vi "comport.vi"() -> ()   [LabVIEW 2022 SP3]
panel:
  in  "COM 6":string
  in  "Refresh Button":bool
  in  "COM 5":string
  in  "COM 4":string
  in  "COM 3":string
  in  "COM 2":string
  out "error out 8":errorcluster
  out "error out 7":errorcluster
  out "error out 6":errorcluster
  out "error out 5":errorcluster
  out "error out 4":errorcluster
  out "error out 3":errorcluster
  out "error out 2":errorcluster
  in  "OK Button":bool
  out "error out":errorcluster
  in  "3":string
  in  "2":string
  in  "1":string
  in  "COM":string
  # "REFERENCE CHECK"
  # "COM A"
  # "COM B"
  # "COM C"
  # "COM D"
  # "Refresh"
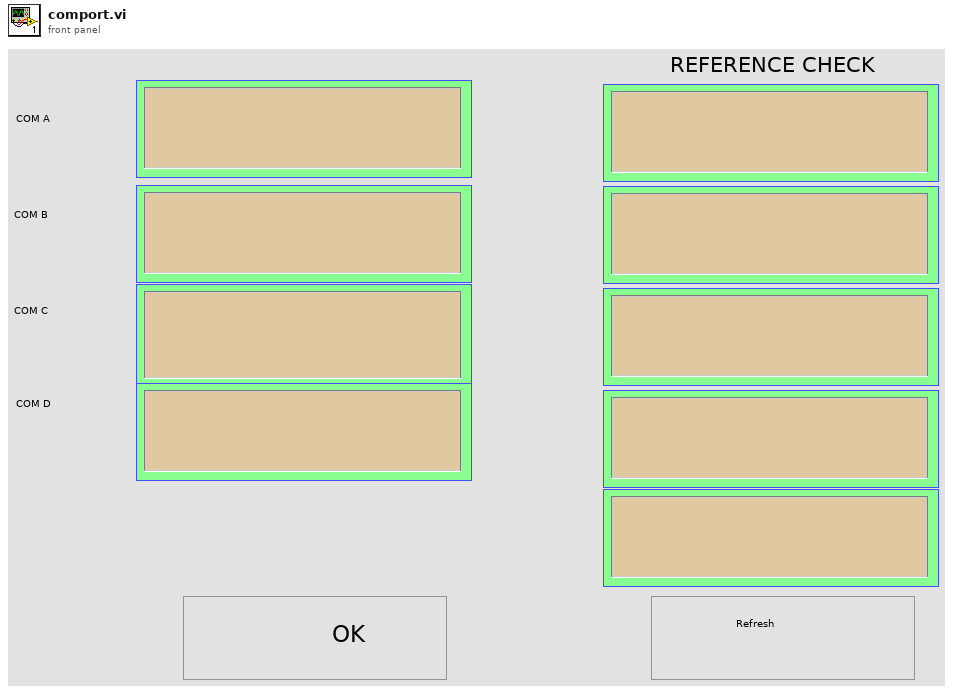
[diagram p1: front panel]
types:
  T1 = enum16{"open", "replace", "create", "open or create", "replace or create", "replace or create with confirmation"}
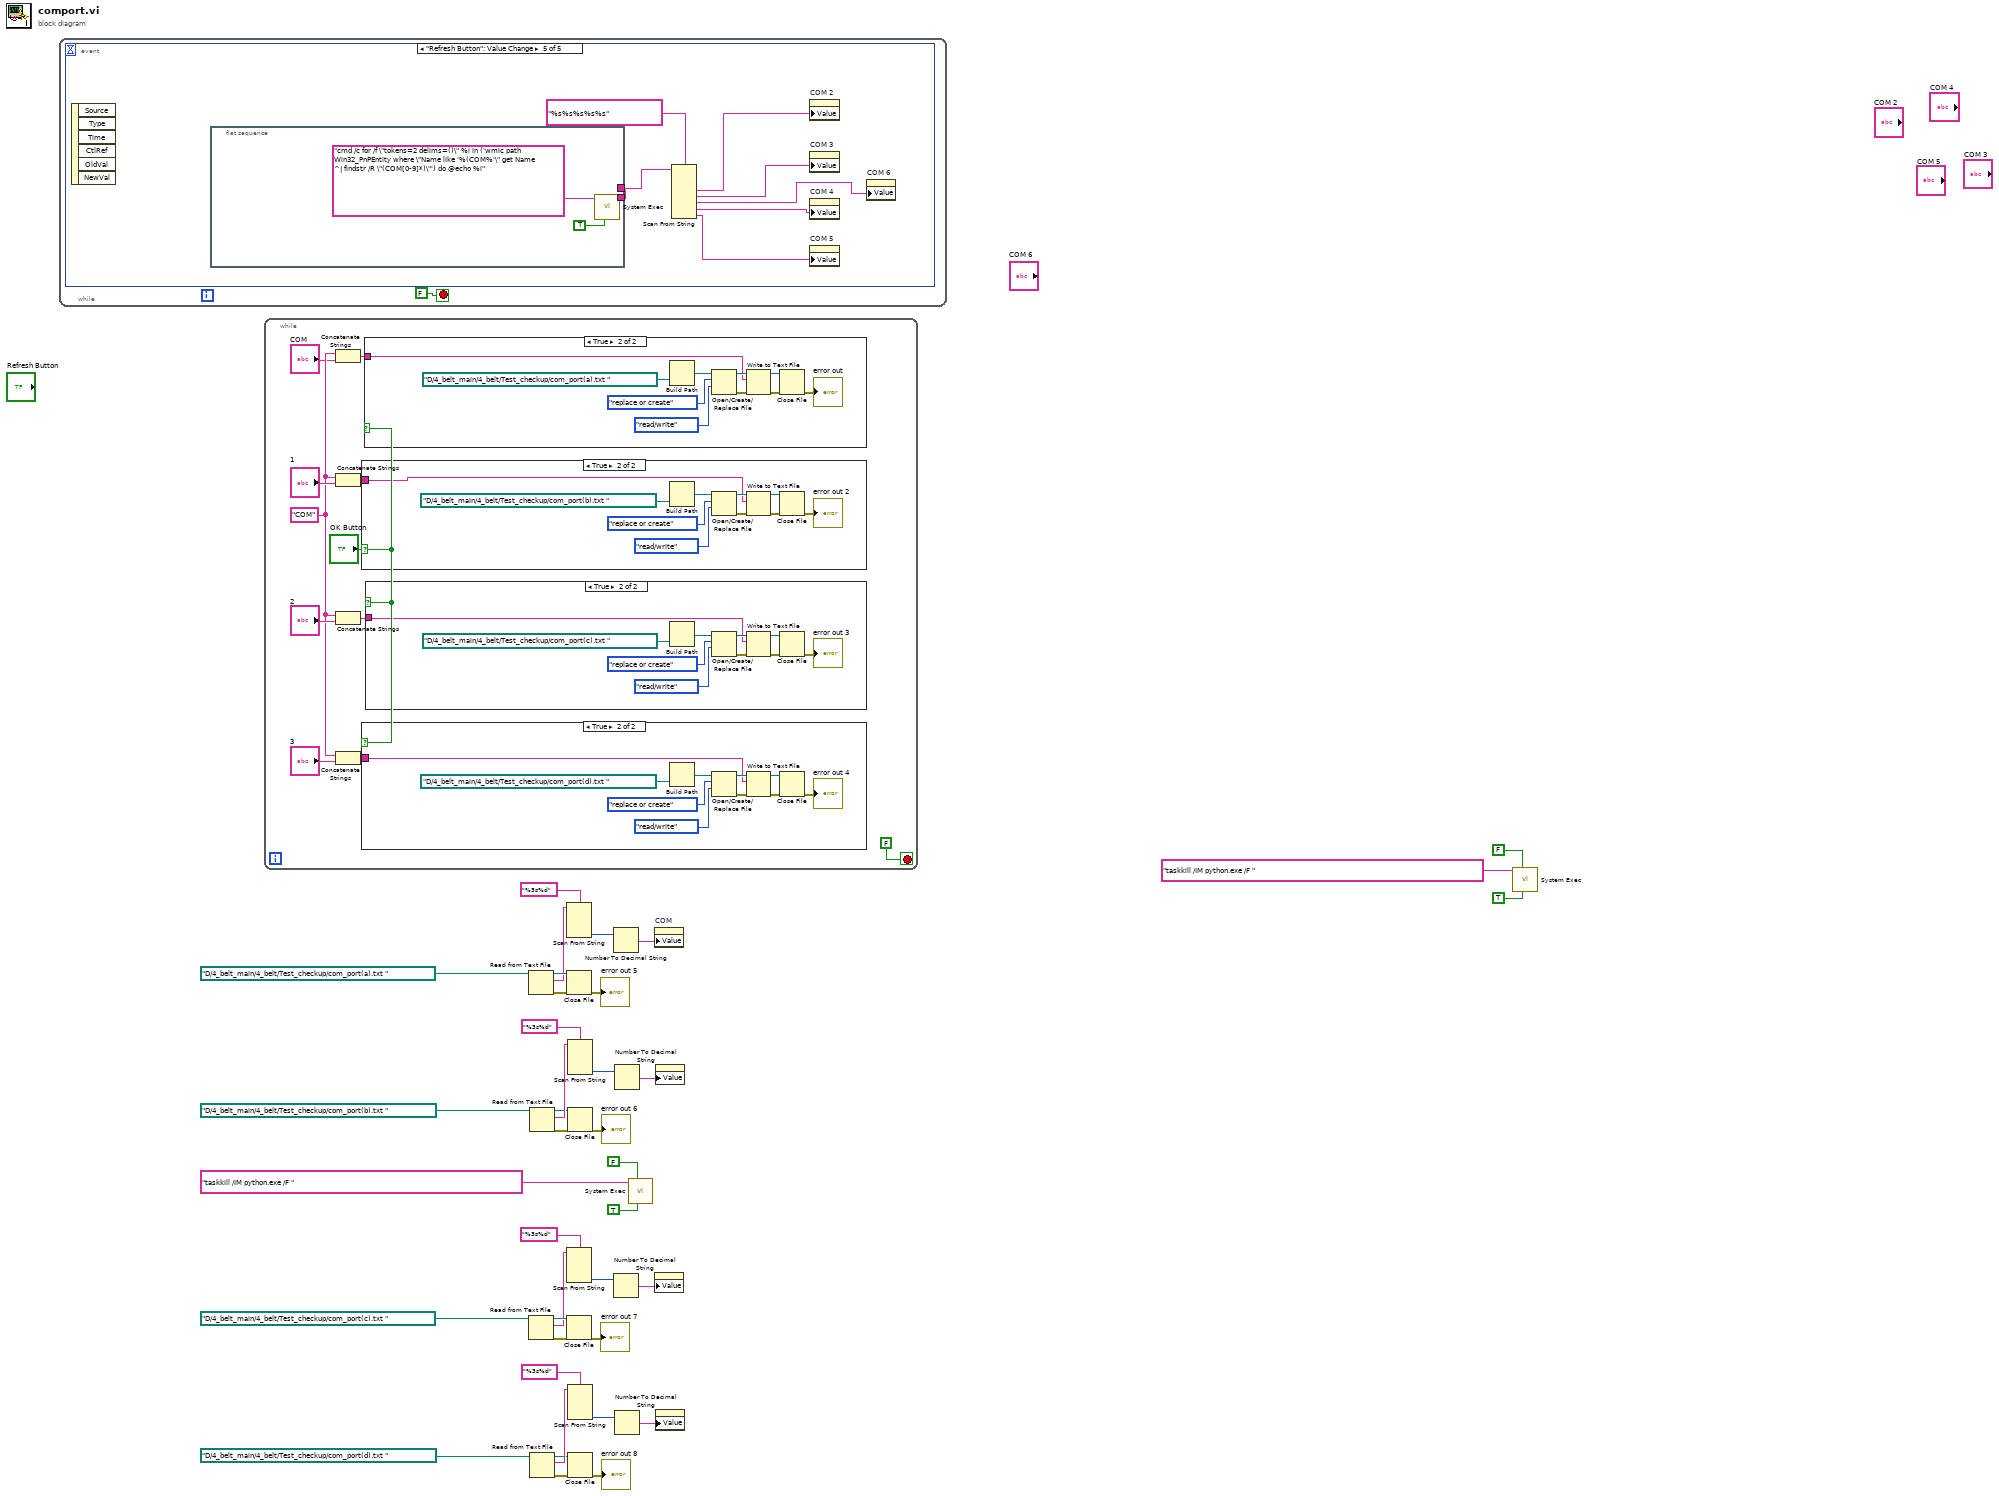
[diagram p0: block diagram]
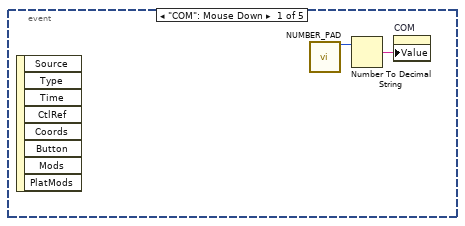
[diagram p2: hidden frame]
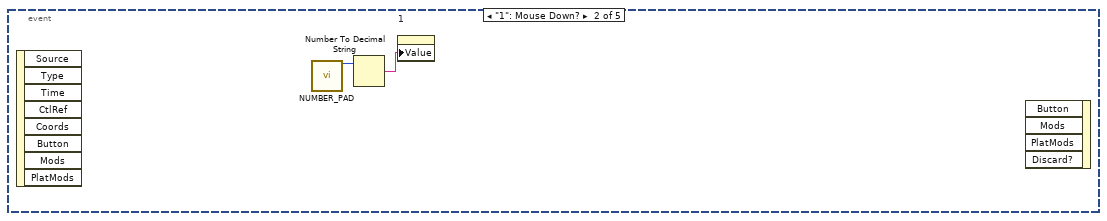
[diagram p3: hidden frame]
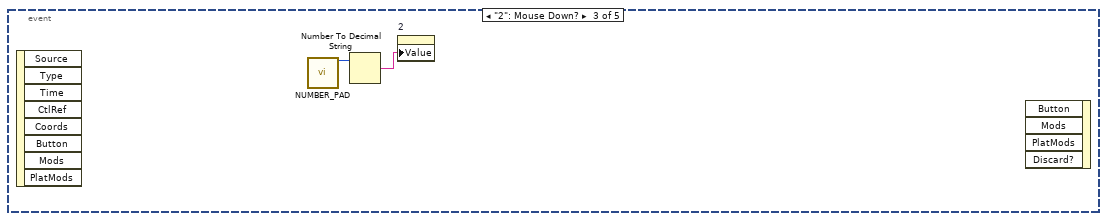
[diagram p4: hidden frame]
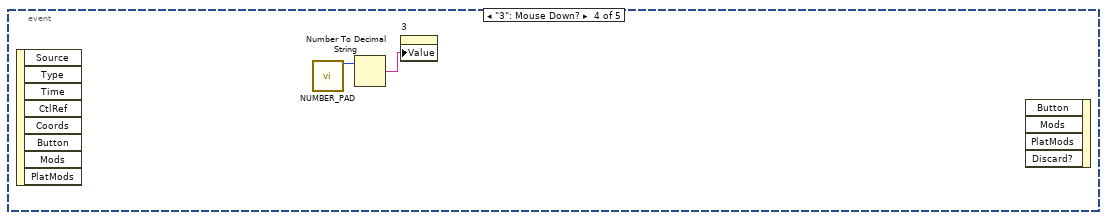
[diagram p5: hidden frame]
diagram:
  n1 = while {
    stop <- FALSE stop-if-true
    n2 = event shown="[4] \"Refresh Button\": Value Change" {
      selector: _ -> [_ _ _ _ _]
      dyn-events: _ -> [_ _ _ _ _]
      timeout: _ -> [_ _ _ _ _]
      event "COM": Mouse Down {
        n3 = event-data() -> ()  [unwired: 1 in, 8 out]
        n4 = call "NUMBER_PAD.vi"() -> ("number (out)"=w41:i32)  [unwired: 15 in]
        n5 = Number To Decimal String(number=w41) -> (decimal integer string=w40:string)  [unwired: 1 in]
        n6 = property on="COM" class="Str"("Value"=w40) -> ()  [unwired: 2 in, 2 out]
      }
      event "1": Mouse Down? {
        n7 = event-data() -> ()  [unwired: 1 in, 8 out]
        n8 = call "NUMBER_PAD.vi"() -> ("number (out)"=w43:i32)  [unwired: 15 in]
        n9 = Number To Decimal String(number=w43) -> (decimal integer string=w42:string)  [unwired: 1 in]
        n10 = property on="1" class="Str"("Value"=w42) -> ()  [unwired: 2 in, 2 out]
        n11 = event-data() -> ()  [unwired: 5 in, 1 out]
      }
      event "2": Mouse Down? {
        n12 = event-data() -> ()  [unwired: 1 in, 8 out]
        n13 = call "NUMBER_PAD.vi"() -> ("number (out)"=w45:i32)  [unwired: 15 in]
        n14 = Number To Decimal String(number=w45) -> (decimal integer string=w44:string)  [unwired: 1 in]
        n15 = property on="2" class="Str"("Value"=w44) -> ()  [unwired: 2 in, 2 out]
        n16 = event-data() -> ()  [unwired: 5 in, 1 out]
      }
      event "3": Mouse Down? {
        n17 = event-data() -> ()  [unwired: 1 in, 8 out]
        n18 = call "NUMBER_PAD.vi"() -> ("number (out)"=w47:i32)  [unwired: 15 in]
        n19 = Number To Decimal String(number=w47) -> (decimal integer string=w46:string)  [unwired: 1 in]
        n20 = property on="3" class="Str"("Value"=w46) -> ()  [unwired: 2 in, 2 out]
        n21 = event-data() -> ()  [unwired: 5 in, 1 out]
      }
      event "Refresh Button": Value Change {
        n22 = event-data() -> ()  [unwired: 1 in, 6 out]
        n23 = flat-sequence {
          tunnel: [w55] -> w52
          tunnel: [w55] -> _
          frame #0 {
            n24 = call <vilib>:"System Exec.vi"("run minimized? (F)"=TRUE, "command line"="cmd /c for /f \"tokens=2 delims=()\" %i in ('wmic path Win32_PnPEntity where \"Name like '%(COM%'\" get Name ^| findstr /R \"(COM[0-9]*)\"') do @echo %i") -> ("standard output"=w55:string)  [unwired: 6 in, 3 out]
          }
        }
        n25 = Scan From String(format string="%s%s%s%s%s", input string=w52) -> (output 1=w50:string, output 2=w49:string, output 3=w48:string, output 4=w53:string, output 5=w54:string)  [unwired: 7 in, 3 out]
        n26 = property on="COM 2" class="Str"("Value"=w50) -> ()  [unwired: 2 in, 2 out]
        n27 = property on="COM 3" class="Str"("Value"=w49) -> ()  [unwired: 2 in, 2 out]
        n28 = property on="COM 4" class="Str"("Value"=w53) -> ()  [unwired: 2 in, 2 out]
        n29 = property on="COM 5" class="Str"("Value"=w54) -> ()  [unwired: 2 in, 2 out]
        n30 = property on="COM 6" class="Str"("Value"=w48) -> ()  [unwired: 2 in, 2 out]
      }
    }
  }
  n31 = while {
    stop <- FALSE stop-if-true
    w65 = "COM"
    n32 = Concatenate Strings(w65, "COM") -> (w64:string)
    n33 = Concatenate Strings(w65, "1") -> (w63:string)
    n34 = Concatenate Strings(w65, "2") -> (w62:string)
    n35 = Concatenate Strings(w65, "3") -> (w61:string)
    n36 = case shown="True" "OK Button" {
      tunnel: w63 -> [_ w90]
      frame False {
      }
      frame True {
        n37 = Build Path(name or relative path=path "D:/4_belt_main/4_belt/Test_checkup/com_port(b).txt " ("base path")) -> (appended path=w98:path)  [unwired: 1 in]
        n38 = Open/Create/Replace File(file path (use dialog)=w98, operation (0:open)=T1."replace or create", access (0:read/write)=enum16{"read/write", "read-only", "write-only"}."read/write") -> (refnum out=w95:refnum<file>, error out=w94:errorcluster)  [unwired: 3 in, 1 out]
        n39 = Write to Text File(file (use dialog)=w95, text=w90, error in=w94) -> (refnum out=w92:refnum<file>, error out=w93:errorcluster)  [unwired: 1 in, 1 out]
        n40 = Close File(refnum=w92, error in=w93) -> (error out=→"error out 2":errorcluster)  [unwired: 1 out]
      }
    }
    n41 = case shown="True" "OK Button" {
      tunnel: w61 -> [_ w70]
      frame False {
      }
      frame True {
        n42 = Build Path(name or relative path=path "D:/4_belt_main/4_belt/Test_checkup/com_port(d).txt " ("base path")) -> (appended path=w78:path)  [unwired: 1 in]
        n43 = Open/Create/Replace File(file path (use dialog)=w78, operation (0:open)=T1."replace or create", access (0:read/write)=enum16{"read/write", "read-only", "write-only"}."read/write") -> (refnum out=w75:refnum<file>, error out=w74:errorcluster)  [unwired: 3 in, 1 out]
        n44 = Write to Text File(file (use dialog)=w75, text=w70, error in=w74) -> (refnum out=w72:refnum<file>, error out=w73:errorcluster)  [unwired: 1 in, 1 out]
        n45 = Close File(refnum=w72, error in=w73) -> (error out=→"error out 4":errorcluster)  [unwired: 1 out]
      }
    }
    n46 = case shown="True" "OK Button" {
      tunnel: w64 -> [_ w100]
      frame False {
      }
      frame True {
        n47 = Build Path(name or relative path=path "D:/4_belt_main/4_belt/Test_checkup/com_port(a).txt " ("base path")) -> (appended path=w108:path)  [unwired: 1 in]
        n48 = Open/Create/Replace File(file path (use dialog)=w108, operation (0:open)=T1."replace or create", access (0:read/write)=enum16{"read/write", "read-only", "write-only"}."read/write") -> (refnum out=w105:refnum<file>, error out=w104:errorcluster)  [unwired: 3 in, 1 out]
        n49 = Write to Text File(file (use dialog)=w105, text=w100, error in=w104) -> (refnum out=w102:refnum<file>, error out=w103:errorcluster)  [unwired: 1 in, 1 out]
        n50 = Close File(refnum=w102, error in=w103) -> (error out=→"error out":errorcluster)  [unwired: 1 out]
      }
    }
    n51 = case shown="True" "OK Button" {
      tunnel: w62 -> [_ w80]
      frame False {
      }
      frame True {
        n52 = Build Path(name or relative path=path "D:/4_belt_main/4_belt/Test_checkup/com_port(c).txt " ("base path")) -> (appended path=w88:path)  [unwired: 1 in]
        n53 = Open/Create/Replace File(file path (use dialog)=w88, operation (0:open)=T1."replace or create", access (0:read/write)=enum16{"read/write", "read-only", "write-only"}."read/write") -> (refnum out=w85:refnum<file>, error out=w84:errorcluster)  [unwired: 3 in, 1 out]
        n54 = Write to Text File(file (use dialog)=w85, text=w80, error in=w84) -> (refnum out=w82:refnum<file>, error out=w83:errorcluster)  [unwired: 1 in, 1 out]
        n55 = Close File(refnum=w82, error in=w83) -> (error out=→"error out 3":errorcluster)  [unwired: 1 out]
      }
    }
  }
  n56 = Read from Text File(file (use dialog)=path "D:/4_belt_main/4_belt/Test_checkup/com_port(a).txt " ("base path")) -> (refnum out=w38:refnum<file>, text=w34:string, error out=w37:errorcluster)  [unwired: 3 in, 1 out]
  n57 = Read from Text File(file (use dialog)=path "D:/4_belt_main/4_belt/Test_checkup/com_port(c).txt " ("base path")) -> (refnum out=w23:refnum<file>, text=w19:string, error out=w22:errorcluster)  [unwired: 3 in, 1 out]
  n58 = Read from Text File(file (use dialog)=path "D:/4_belt_main/4_belt/Test_checkup/com_port(b).txt " ("base path")) -> (refnum out=w24:refnum<file>, text=w28:string, error out=w25:errorcluster)  [unwired: 3 in, 1 out]
  n59 = Read from Text File(file (use dialog)=path "D:/4_belt_main/4_belt/Test_checkup/com_port(d).txt " ("base path")) -> (refnum out=w10:refnum<file>, text=w14:string, error out=w11:errorcluster)  [unwired: 3 in, 1 out]
  n60 = Scan From String(format string="%3s%d", input string=w34) -> (output 2=w32:i32)  [unwired: 5 in, 3 out]
  n61 = Close File(refnum=w38, error in=w37) -> (error out=→"error out 5":errorcluster)  [unwired: 1 out]
  n62 = Scan From String(format string="%3s%d", input string=w19) -> (output 2=w17:i32)  [unwired: 5 in, 3 out]
  n63 = Close File(refnum=w23, error in=w22) -> (error out=→"error out 7":errorcluster)  [unwired: 1 out]
  n64 = Scan From String(format string="%3s%d", input string=w28) -> (output 2=w30:i32)  [unwired: 5 in, 3 out]
  n65 = Close File(refnum=w24, error in=w25) -> (error out=→"error out 6":errorcluster)  [unwired: 1 out]
  n66 = Scan From String(format string="%3s%d", input string=w14) -> (output 2=w16:i32)  [unwired: 5 in, 3 out]
  n67 = Close File(refnum=w10, error in=w11) -> (error out=→"error out 8":errorcluster)  [unwired: 1 out]
  n68 = Number To Decimal String(number=w32) -> (decimal integer string=w31:string)  [unwired: 1 in]
  n69 = Number To Decimal String(number=w17) -> (decimal integer string=w8:string)  [unwired: 1 in]
  n70 = Number To Decimal String(number=w30) -> (decimal integer string=w9:string)  [unwired: 1 in]
  n71 = Number To Decimal String(number=w16) -> (decimal integer string=w7:string)  [unwired: 1 in]
  n72 = call <vilib>:"System Exec.vi"("run minimized? (F)"=TRUE, "wait until completion? (T)"=FALSE, "command line"="taskkill /IM python.exe /F ") -> ()  [unwired: 5 in, 4 out]
  n73 = property on="COM" class="Str"("Value"=w31) -> ()  [unwired: 2 in, 2 out]
  n74 = property on="2" class="Str"("Value"=w8) -> ()  [unwired: 2 in, 2 out]
  n75 = property on="1" class="Str"("Value"=w9) -> ()  [unwired: 2 in, 2 out]
  n76 = property on="3" class="Str"("Value"=w7) -> ()  [unwired: 2 in, 2 out]
  n77 = call <vilib>:"System Exec.vi"("run minimized? (F)"=TRUE, "wait until completion? (T)"=FALSE, "command line"="taskkill /IM python.exe /F ") -> ()  [unwired: 5 in, 4 out]
